vi "SearchSpecialChar.vi"(1 "正则表达式":string) -> (0 "字符串":string)   [LabVIEW 2013]
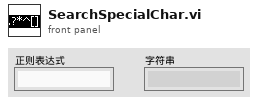
[diagram p1: front panel]
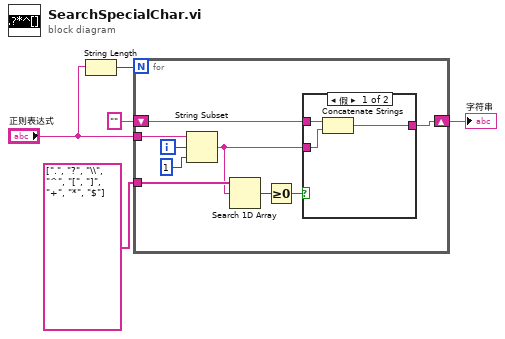
[diagram p0: block diagram]
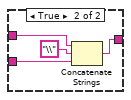
[diagram p2: hidden frame]
diagram:
  n1 = String Length(string="正则表达式") -> (length=w3:i32)
  n2 = for {
    N: w3 -> [_]
    tunnel: "正则表达式" -> [w14]
    tunnel: string[] [".", "?", "\\", "^", "[", "]", "+", "*", "$"] ("一维数组") -> [w11]
    shift-right: [w9] -> w5
    shift-left: "" -> [w8]
    i -> [w13]
    n3 = String Subset(string=w14, offset (0)=w13, length (rest)=1 ("长度（剩余）")) -> (substring=w6:string)
    n4 = Search 1D Array(1D array=w11, element=w6) -> (index of element=w10:i32)  [unwired: 1 in]
    n5 = Greater Or Equal To 0?(x=w10) -> (x >= 0?=w7:bool)
    n6 = case shown="假" w7 {
      tunnel: [w15 w21] -> w9
      tunnel: w8 -> [w17 w20]
      tunnel: w6 -> [w16 w18]
      frame False {
        n7 = Concatenate Strings(w17, w16) -> (w15:string)
      }
      frame True {
        n8 = Concatenate Strings(w20, "\\" ("字符串"), w18) -> (w21:string)
      }
    }
  }
  "字符串" <- w5
